vi "Handle Last Ack Core.vi"(4 "error in (no error)":errorcluster, 6 "Last Ack":refnum<class "Last Ack.lvclass">, 7 "HIJ Vision Camera App in":refnum<class "HIJ Vision Camera App.lvclass">) -> (0 "error out":errorcluster, 3 "HIJ Vision Camera App out":refnum<class "HIJ Vision Camera App.lvclass">)   [LabVIEW 2020, in "HIJ Vision Camera App.lvlib" / "HIJ Vision Camera App.lvclass"]
doc: "(<B>Filename</B>: Actor Framework.lvlib:Actor.lvclass:Handle Last Ack Core.vi)\n\nDefines how the caller actor responds to the Last Ack message from a nested actor. The Last Ack message is the final message a nested actor sends to its caller before it shuts down. The message contains information about the final state of the nested actor.\n\nBy default, this method does nothing except return any error the nested actor sent. A descendant class may override this method to define behavior."
uses:
  HIJ Vision Camera App.lvclass
  <vilib>/ActorFramework/LastAck/Last Ack.lvclass
  HIJ Vision Camera App Dialog/HIJ Vision Camera App Dialog/HIJ Vision Camera App Dialog.lvclass
  <vilib>/ActorFramework/LastAck/Last Ack.lvclass/Last Ack.ctl
  <vilib>/ActorFramework/Message Enqueuer/Message Enqueuer.lvclass
  HIJ Vision Camera App.lvclass/HIJ Vision Camera App.ctl
  HIJ Vision Application/HIJ Vision Application/HIJ Vision Application.lvclass
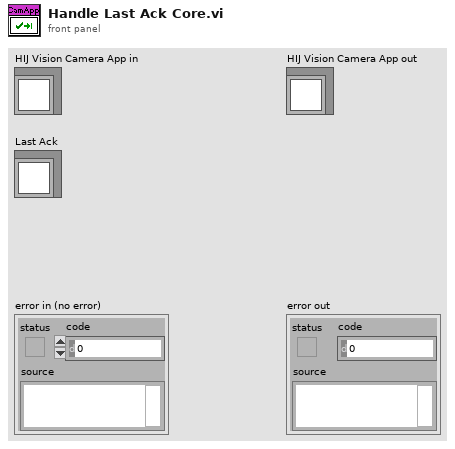
[diagram p1: front panel]
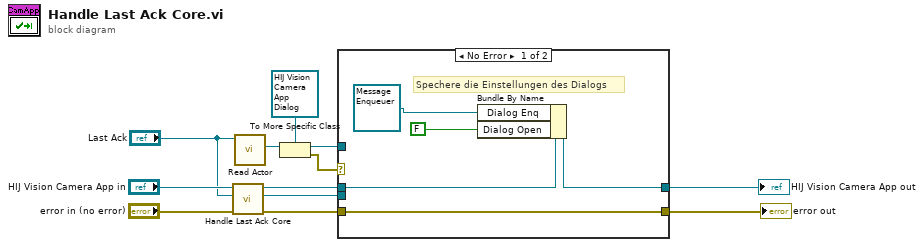
[diagram p0: block diagram]
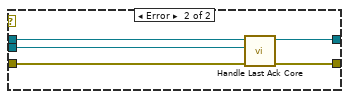
[diagram p2: hidden frame]
diagram:
  n1 = call-parent "Handle Last Ack Core.vi"("error in (no error)"="error in (no error)", "Last Ack"="Last Ack", "ViewableActor in"="HIJ Vision Camera App in") -> ("error out"=w2:errorcluster, "ViewableActor out"=w4:refnum<class "HIJ Vision Camera App.lvclass">)  [unwired: 3 in]
  n2 = call <vilib>:"Read Actor.vi"("Last Ack"="Last Ack") -> ("Actor"=w7:refnum<class "Actor.lvclass">)  [unwired: 10 in]
  n3 = To More Specific Class(target class=refnum<class "HIJ Vision Camera App Dialog.lvclass"> refnum ("HIJ Vision Camera App Dialog.lvlib:HIJ Vision Camera App Dialog.lvclass"), reference=w7) -> (specific class reference=w6:refnum<class "HIJ Vision Camera App Dialog.lvclass">, error out=w5:errorcluster)  [unwired: 1 in]
  n4 = case shown="No Error" w5 {
    tunnel: [w16 w21] -> w11
    tunnel: [w14 w20] -> w10
    tunnel: w2 -> [w16 w19]
    tunnel: w4 -> [w15 w18]
    tunnel: "Last Ack" -> [_ w17]
    tunnel: w6 -> [_ _]
    frame No Error {
      # "Spechere die Einstellungen des Dialogs"
      n5 = Bundle By Name(cluster=w15, "Dialog Enq"=refnum<class "Message Enqueuer.lvclass"> refnum, "Dialog Open"=FALSE) -> (w14:refnum<class "HIJ Vision Camera App.lvclass">)
    }
    frame Error {
      n6 = call-parent "Handle Last Ack Core.vi"("error in (no error)"=w19, "Last Ack"=w17, "ViewableActor in"=w18) -> ("error out"=w21:errorcluster, "ViewableActor out"=w20:refnum<class "HIJ Vision Camera App.lvclass">)  [unwired: 3 in]
    }
  }
  "HIJ Vision Camera App out" <- w10
  "error out" <- w11
